vi "CO2 Actor Send Error Report.vi"(7 "Message Priority (Normal)":T1=enum."Normal", 8 "Error From Sender":errorcluster, 11 "CO2 Actor in":refnum<class "CO2 Actor.lvclass">) -> (3 "CO2 Actor out":refnum<class "CO2 Actor.lvclass">)   [LabVIEW 2015, in "cRIO-Carbondioxide.lvlib" / "CO2-Actor.lvlib" / "CO2 Actor.lvclass"]
uses:
  CO2 Actor.lvclass
  <vilib>/ActorFramework/Message Enqueuer/Message Priority.ctl
  <vilib>/ActorFramework/Actor/Actor.lvclass/Actor.ctl
  <vilib>/ActorFramework/Message Enqueuer/Message Enqueuer.lvclass/Message Enqueuer.ctl
  <vilib>/ActorFramework/Report Error Msg/Report Error Msg.lvclass/Report Error Msg.ctl
  <vilib>/ActorFramework/Message Enqueuer/Enqueue.vi
  <vilib>/ActorFramework/Actor/Read Self Enqueuer.vi
  <vilib>/ActorFramework/Message Enqueuer/Init from Existing Queue.vi
  <vilib>/ActorFramework/Message Priority Queue/Priority Enqueue.vi
  <vilib>/ActorFramework/Report Error Msg/Report Error Msg.lvclass
  <vilib>/ActorFramework/Message Enqueuer/Message Enqueuer.lvclass
  <vilib>/ActorFramework/Actor/Actor.lvclass
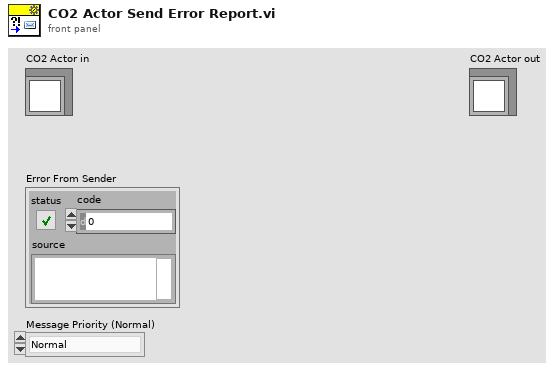
[diagram p1: front panel]
types:
  T1 = typedef "Actor Framework.lvlib/Message Enqueuer.lvclass/Message Priority.ctl" = enum16{"Low", "Normal", "High"}
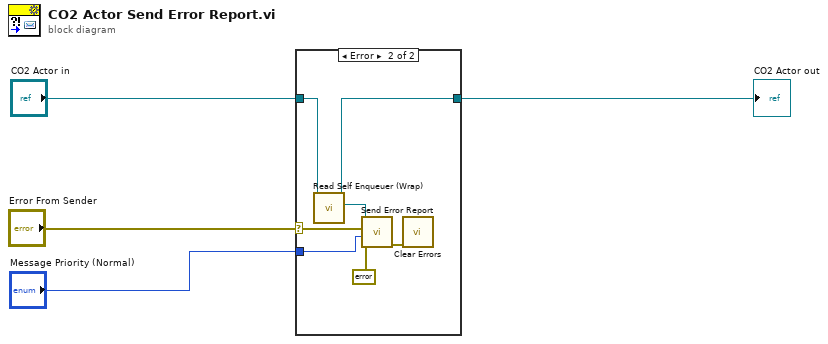
[diagram p0: block diagram]
diagram:
  n1 = case shown="Error" "Error From Sender" {
    selector: "Error From Sender" -> [_ w11]
    tunnel: "CO2 Actor in" -> [w5 w7]
    tunnel: [w5 w8] -> w2
    tunnel: "Message Priority (Normal)" -> [_ w6]
    frame No Error {
    }
    frame Error {
      n2 = call "Read Self Enqueuer (Wrap).vi"("CO2 Actor in"=w7) -> ("Actor Framework:Message Enqueuer"=w10:refnum<class "Message Enqueuer.lvclass">, "CO2 Actor out"=w8:refnum<class "CO2 Actor.lvclass">)  [unwired: 9 in]
      n3 = call <vilib>:"Send Error Report.vi"("error in (no error)"=errorcluster {"status"=FALSE, "code"=0, "source"=""}, "Message Priority (Normal)"=w6, "Error From Sender"=w11, "Message Enqueuer"=w10) -> ("error out"=w9:errorcluster)  [unwired: 7 in]
      n4 = call <vilib>:"Clear Errors.vi"("error in (no error)"=w9) -> ()  [unwired: 5 in, 2 out]
    }
  }
  "CO2 Actor out" <- w2
